vi "MISC High Res Time.vi"(7 "Time Standard (am/pm)":enum16{"AM/PM", "24 Hour"}(ring), 8 "Date Format (Abb)":enum16{"short", "long", "abbreviated"}(ring)=enum."abbreviated", 9 "Mode (add date)":enum16{"Add Date", "Time Only"}(ring)) -> (1 "Date/Time String":string)   [LabVIEW 2017]
doc: "This VI simply returns a formatted string containing the current date and time to the resolution of 0.001-seconds.\n\nFrom the inputs the date format can be changed and the time standard can be chosen (24Hour or AM/PM).\n\nThis vi was created by David Gianetto, contact me with any problems, questions, etc."
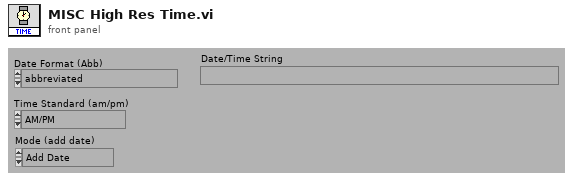
[diagram p1: front panel]
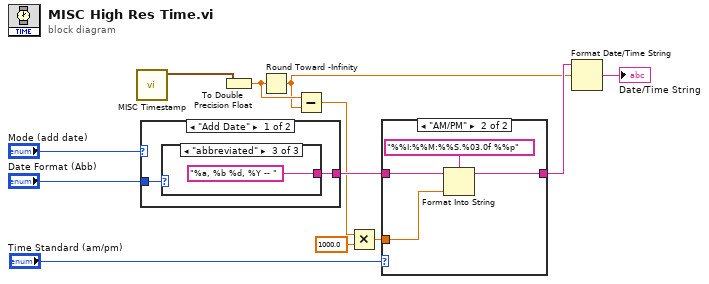
[diagram p0: block diagram]
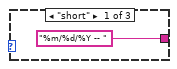
[diagram p2: hidden frame]
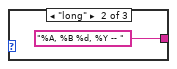
[diagram p3: hidden frame]
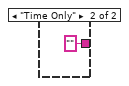
[diagram p4: hidden frame]
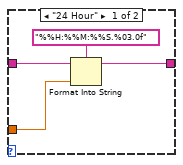
[diagram p5: hidden frame]
diagram:
  n1 = call "MISC Timestamp.vi"() -> ("Timestamp"=w1:timestamp)  [unwired: 1 in, 10 out]
  n2 = case shown="\"Add Date\"" "Mode (add date)" {
    tunnel: "Date Format (Abb)" -> [w14 _]
    tunnel: [w13 ""] -> w9
    frame "Add Date" {
      n3 = case shown="\"abbreviated\"" w14 {
        tunnel: ["%m/%d/%Y -- " "%A, %B %d, %Y -- " "%a, %b %d, %Y -- "] -> w13
        frame "short" {
        }
        frame "long" {
        }
        frame "abbreviated" {
        }
      }
    }
    frame "Time Only" {
    }
  }
  n4 = To Double Precision Float(number=w1) -> (double precision float=w12:dbl)
  n5 = Round Toward -Infinity(1:w12) -> (0:w4:dbl)
  n6 = Subtract(x=w12, y=w4) -> (x-y=w3:dbl)
  n7 = Multiply(x=w3, y=1000.0) -> (x*y=w7:dbl)
  n8 = case shown="\"AM/PM\"" "Time Standard (am/pm)" {
    tunnel: w9 -> [w21 w25]
    tunnel: w7 -> [w22 w26]
    tunnel: [w19 w23] -> w6
    frame "24 Hour" {
      n9 = Format Into String(format string="%%H:%%M:%%S.%03.0f" ("Format String"), initial string=w21, w22) -> (resulting string=w19:string)  [unwired: 1 in, 1 out]
    }
    frame "AM/PM" {
      n10 = Format Into String(format string="%%I:%%M:%%S.%03.0f %%p" ("Format String"), initial string=w25, w26) -> (resulting string=w23:string)  [unwired: 1 in, 1 out]
    }
  }
  n11 = Format Date/Time String(time format string (%c)=w6, seconds (now)=w4) -> (date/time string=→"Date/Time String":string)  [unwired: 1 out]
